vi "write Double.vi"(9 "value":dbl, 10 "index":i32, 11 "data table in":T1) -> (3 "data table out":T1)   [LabVIEW 2013, in "data bus values.lvlib"]
doc: "Writes a single value to the data table."
uses:
  data bus values.lvlib
  data table.ctl
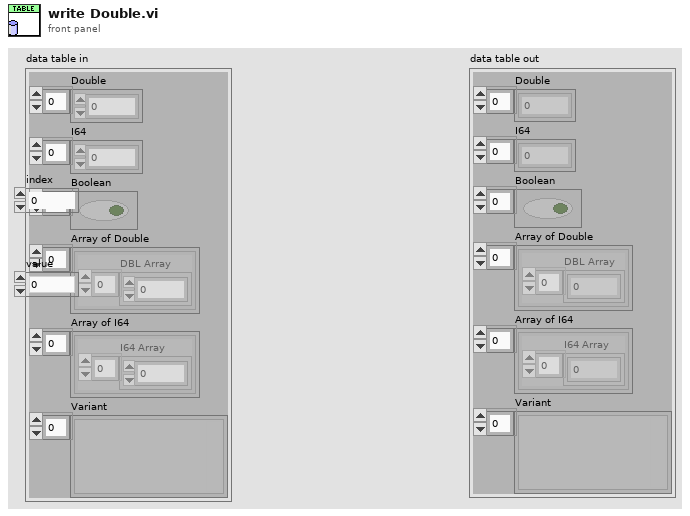
[diagram p1: front panel]
types:
  T1 = typedef "data bus values.lvlib/data table.ctl" = cluster{"Double":dbl[], "I64":i64[], "Boolean":bool[], "Array of Double":cluster{"DBL Array":dbl[]}[], "Array of I64":cluster{"I64 Array":i64[]}[], "Variant":variant[]}
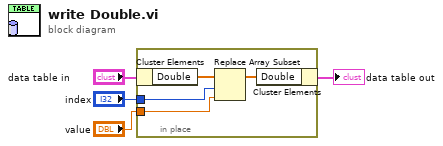
[diagram p0: block diagram]
diagram:
  n1 = in-place {
    in-place-border: "index" -> [w8]
    in-place-border: "value" -> [w7]
    n2 = in-place-cluster #1("data table in") -> ("Double"=w6:dbl[])
    n3 = Replace Array Subset(array=w6, new element=w7, index=w8) -> (w5:dbl[])
    n4 = in-place-cluster #1("Double"=w5) -> (→"data table out":T1)
  }
